vi "BotSpeak_DebugScript.vi"(2 "Subroutine (runs prgm if unwired)":string, 3 "Bot Settings":T1) -> (0 "response":string="169.254.32.85", 1 "Bot Settings":T1)   [LabVIEW 2014]
doc: "Runs scripted code in debug mode."
uses:
  <userlib>/botspeak/VIs/Direct/BotSpeak_Control.ctl
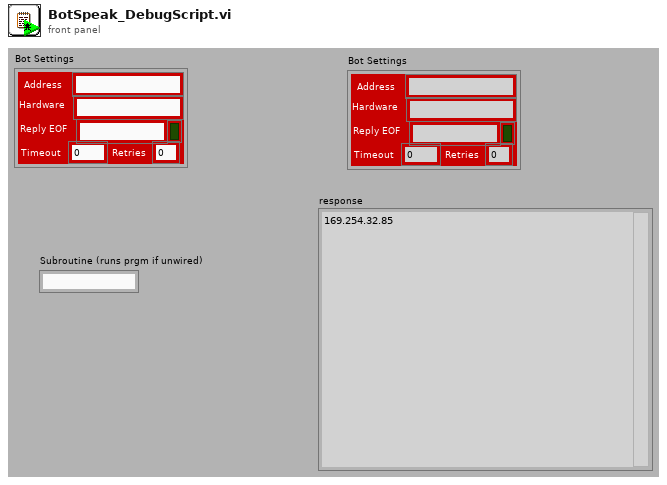
[diagram p1: front panel]
types:
  T1 = typedef "BotSpeak_Control.ctl" = cluster{"Address":string, "Reply EOF":string, "Hardware":string, "Retries":i8, "Timeout":i32, "Open?":bool}
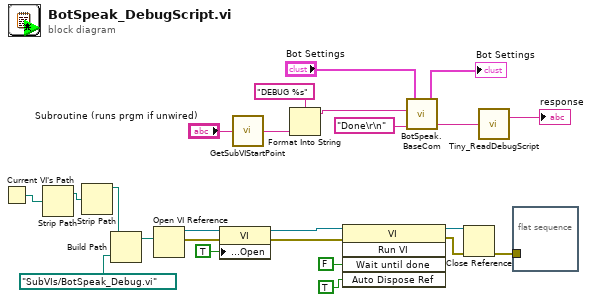
[diagram p0: block diagram]
diagram:
  n1 = Current VI's Path() -> (path=w21:path)
  n2 = Strip Path(path=w21) -> (stripped path=w9:path)  [unwired: 1 out]
  n3 = Strip Path(path=w9) -> (stripped path=w8:path)  [unwired: 1 out]
  n4 = Build Path(base path=w8, name or relative path=path "SubVIs/BotSpeak_Debug.vi") -> (appended path=w19:path)
  n5 = Open VI Reference(vi path=w19) -> (vi reference=w18:refnum<vi>, error out=w11:errorcluster)  [unwired: 5 in]
  n6 = property class="VI"(reference=w18, error in=w11, "Front Panel.Open"=TRUE ("Front Panel Window:Open")) -> (reference out=w13:refnum<vi>, error out=w10:errorcluster)
  n7 = call <userlib>:"GetSubVIStartPoint.vi"("Subroutine (runs prgm if unwired)"="Subroutine (runs prgm if unwired)") -> ("String"=w2:string)
  n8 = Format Into String(format string="DEBUG %s" ("command"), w2) -> (resulting string=w1:string)  [unwired: 2 in, 1 out]
  n9 = invoke class="VI" method="Run VI"(reference=w13, error in=w10, "Wait until done"=FALSE ("Wait Until Done"), "Auto Dispose Ref"=TRUE ("Wait Until Done")) -> (reference out=w16:refnum<vi>, error out=w17:errorcluster)  [unwired: 1 in, 3 out]
  n10 = call <userlib>:"BotSpeak.BaseCom.vi"("Termination"="Done\r\n", "command"=w1, "Bot Settings in"="Bot Settings") -> ("response"=w6:string, "Bot Settings out"=→"Bot Settings":T1)  [unwired: 2 in]
  n11 = Close Reference(reference=w16, error in (no error)=w17) -> (error out=w7:errorcluster)
  n12 = call <userlib>:"Tiny_ReadDebugScript.vi"("read buffer"=w6) -> ("read buffer"=→"response":string)  [unwired: 2 in]
  n13 = flat-sequence {
    tunnel: w7 -> [_]
    frame #0 {
    }
  }
